vi "Get SV info.vi"(8 "Error In":errorcluster, 11 "container refnum in":refnum<k21>="ni.var.psp://localhost") -> (0 "Error Out":errorcluster, 2 "Number of Variables":i32, 3 "Deployed Shared Variable Information":T1)   [LabVIEW 2014]
doc: "<B>Copyright</B>: (c) 2015 MHWirth. All rights reserved.\n\nThis SubVI gets all the shared variables deployed on the given container, and provides information associated to the shared variables.\n\nInformation for every shared variable:\n- URL\n- Variable/Parent Name\n- Type"
uses:
  <resource>/objmgr/ni.var.rc
panel:
  out "Data Type Array (String)":string[](array[string])
  out "Variable/Parent Name array":string[][](array[string])
  out "URL array":string[](array[string])
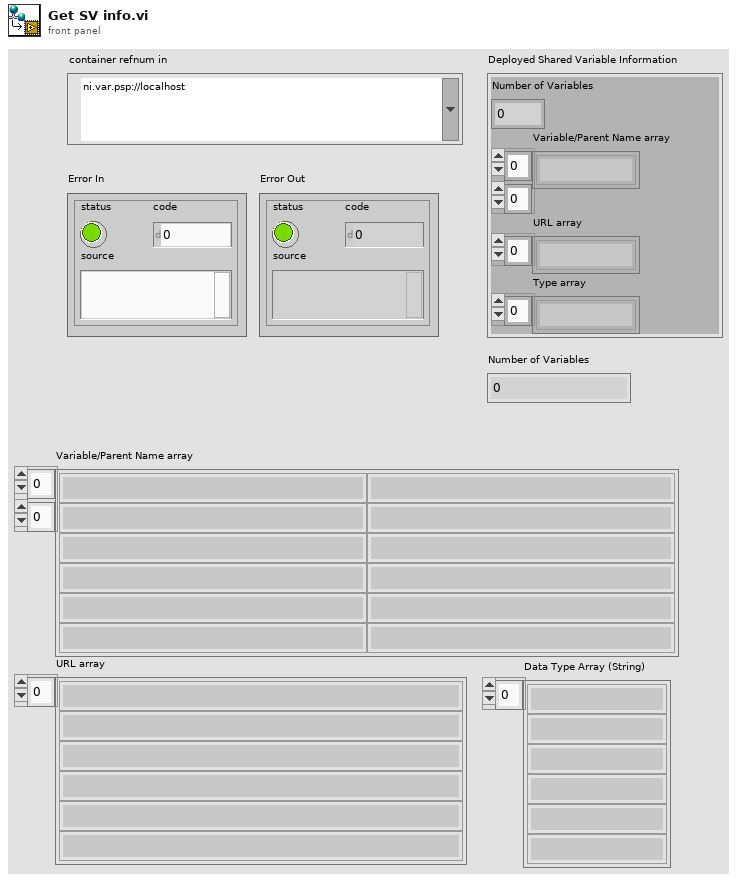
[diagram p1: front panel]
types:
  T1 = cluster{"Number of Variables":i32, "Variable/Parent Name array":string[][], "URL array":string[], "Type array":string[]}
  T2 = cluster{i32, string[][], string[], "Type array":string[]}
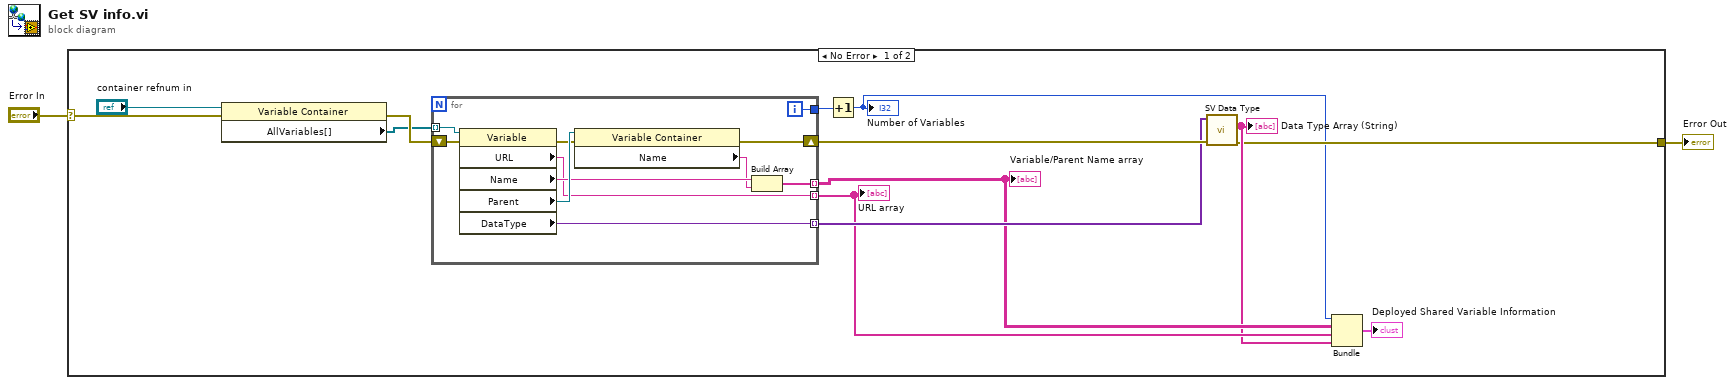
[diagram p0: block diagram]
diagram:
  n1 = case shown="No Error" "Error In" {
    selector: "Error In" -> [w14 w27]
    tunnel: [w5 w27] -> w1
    frame No Error {
      n2 = property class="Variable Container"(reference="container refnum in", error in=w14) -> (error out=w13:errorcluster, "AllVariables[]"=w12:refnum<k21>[])  [unwired: 1 out]
      n3 = for {
        shift-right: [w22] -> w11
        shift-left: w13 -> [w25]
        tunnel: w12 -> [w26] mode=indexing
        tunnel: [w19] -> w9 mode=indexing
        tunnel: [w16] -> w10 mode=indexing
        tunnel: [w18] -> w4
        tunnel: [w17] -> w8 mode=indexing
        i -> [w18]
        n4 = property class="Variable"(reference=w26, error in=w25) -> (error out=w23:errorcluster, "URL"=w17:string, "Name"=w21:string, "Parent"=w24:refnum<k21>, "DataType"=w16:variant)  [unwired: 1 out]
        n5 = property class="Variable Container"(reference=w24, error in=w23) -> (error out=w22:errorcluster, "Name"=w20:string)  [unwired: 1 out]
        n6 = Build Array(w21, w20) -> (w19:string[])
      }
      "URL array" <- w8
      "Variable/Parent Name array" <- w9
      n7 = Increment(x=w4) -> (x+1=w3:i32)
      "Number of Variables" <- w3
      n8 = call "SV Data Type.vi"("Error In"=w11, "Data Type - Variant"=w10) -> ("Error Out"=w5:errorcluster, "Type array"=w7:string[])  [unwired: 7 in, 1 out]
      "Data Type Array (String)" <- w7
      n9 = Bundle(w3, w9, w8, "Type array"=w7) -> (→"Deployed Shared Variable Information":T2)  [unwired: 1 in]
    }
    frame Error {
    }
  }
  "Error Out" <- w1
